vi "Rotate Coordinates.vi"(8 "error in (no error)":errorcluster, 9 "Theta":dbl, 10 "XY In":dbl[](array[numeric]), 11 "Dispense in":refnum<class "Dispense.lvclass">) -> (0 "error out":errorcluster, 2 "XY Out":dbl[](array[numeric]), 3 "Dispense out":refnum<class "Dispense.lvclass">)   [LabVIEW 2021, in "Dispense.lvclass"]
uses:
  Dispense.lvclass
  <vilib>/Analysis/coordinate.llb/2D Cartesian Coordinate Rotation (Scalar).vi
  <vilib>/Analysis/NI_AALPro.lvlib
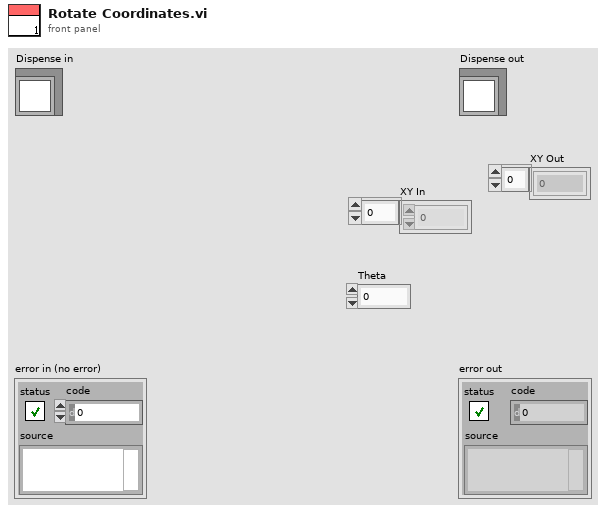
[diagram p1: front panel]
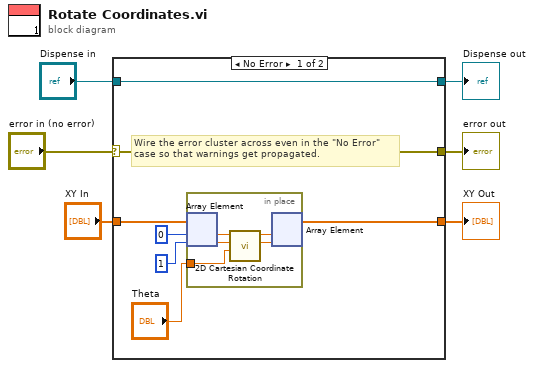
[diagram p0: block diagram]
diagram:
  n1 = case shown="No Error" "error in (no error)" {
    selector: "error in (no error)" -> [w12 w21]
    tunnel: [w12 w21] -> w5
    tunnel: [w13 w20] -> w3
    tunnel: "Dispense in" -> [w13 w20]
    tunnel: [w8 w19] -> w2
    tunnel: "XY In" -> [w7 w19]
    frame No Error {
      # "Wire the error cluster across even in the \"No Error\"\ncase so that warnings get propagated."
      n2 = in-place {
        in-place-border: "Theta" -> [w16]
        n3 = in-place-array #1(w7, 0, 1) -> (w18:dbl, w17:dbl)
        n4 = call-poly <vilib>:"2D Cartesian Coordinate Rotation.vi"("theta"=w16, "y"=w17, "x"=w18) -> ("y out"=w14:dbl, "x out"=w15:dbl)  [unwired: 6 in, 1 out]
        n5 = in-place-array #1(w15, w14) -> (w8:dbl[])  [unwired: 2 out]
      }
    }
    frame Error {
    }
  }
  "error out" <- w5
  "Dispense out" <- w3
  "XY Out" <- w2
